vi "UHR-Fleezers Control (host) - 12.5.vi"() -> ()   [LabVIEW 2012] (continued)
  out "error out":errorcluster
  out "error out 2":errorcluster
  in  "Bottom  1 Harvard Syringe Pump Serial Port":refnum<visa-resource-name>="Bottom-Pump1-COM5"
  in  "Center Harvard Syringe Pump Serial Port":refnum<visa-resource-name>="Central-Pump2-COM6"
  in  "Lost Tether Alarm Threshold (pN)":dbl=0.5
  in  "AOM X Cal (nm/MHz)":dbl=155.0
  in  "MCL X Cal (nm/V)":dbl=1070.0
  out "X RF Amplitude Limits (%)":T16={"Minimum"=0.0, "Maximum"=50.0, "Increment"=1.0}
  out "X RF Frequency Limits (MHz)":T16={"Minimum"=60.0, "Maximum"=90.0, "Increment"=1.0}
  out "Y RF Frequency Limits (MHz)":T16={"Minimum"=0.0, "Maximum"=40.0, "Increment"=1.0}
  out "Y RF Amplitude Limits (%)":T16={"Minimum"=0.0, "Maximum"=50.0, "Increment"=1.0}
  in  "Manip. X?":bool=TRUE
  in  "Manip. Y?":bool
  in  "Force Manip Abort":bool
  out "Read cal error":errorcluster
  in  "DAQ Delay (ms)":u32=1000
  in  "Start Scan":bool
  in  "Scan axis":bool=TRUE
  in  "Osc. amp. (V)":dbl=5.0
  in  "Osc. center (V)":dbl=5.0
  in  "Osc. freq. (Hz) 2":dbl=1.0
  in  "MCL Mode":u16(ring) items=["Manual Positioning", "Sinusoidal Wave", "Linear Scan"]
  in  "Begin (V)":dbl
  in  "End (V)":dbl=10.0
  in  "N Points":dbl=20.0
  in  "Delay to Interlace (s)":dbl
  in  "Delayed Interlace Start":bool
  in  "Read Lateness and Rel Phase":bool=TRUE
  out "Vec Mean of T1 T2":dbl[](array[numeric])=[nan, nan]
  in  "Cal read wait (s)":u32=5
  out "Time tether formed":timestamp=timestamp(3419012832.6319866 s since 1904-01-01)
  in  "Sample Chamber Stage Serial Port":refnum<visa-resource-name>="Sample-Stage-COM1"
  in  "Chemyx Syringe Pump Serial Port":refnum<visa-resource-name>="ASRL3::INSTR"
  in  "Limit Min (MHz)":dbl=10.0 caption="Min (MHz)"
  in  "Limit Max (MHz)":dbl=16.0 caption="Max (MHz)"
  in  "Limits Enable":bool=TRUE caption="Enable"
  out "AI labels":string[](array[string])=["T1 Y", "T1 X", "T1 Sum", "T2 Y", "T2 X", "T2 Sum", "T1 FB X", "T1 FB Sum", "T2 FB X", "T2 FB Sum", "PSD Y", "PSD X", "PSD Y Sum"]
  in  "Save Trap Pos. Data":bool=TRUE
  in  "Lower Ch. Cap.":bool
  in  "Top 3 Harvard Syringe Pump Serial Port":refnum<visa-resource-name>="Top-Pump3-COM4"
  out "Database link":path
  out "connection reference":T17
  # "External fluorescence triggering tests:"
  # "After"
  # "During"
  # "Trap On?"
  # "BD Flow ON?"
  # "Samp Flow ON?"
  # "Trap Trig. Fl.?"
  # "Zero It"
  # "Floor it\n(e.g., hp unwinding)"
  # "1"
  # "2"
  # "Fl. Down"
  # "Fl. Up"
  # "Bead sep"
  # "Trap Display:"
  # "APD Display:"
  # "Data Saving"
  # "DAQ"
  # "Trap Manipulation"
  # "Bead Calibration"
  # "Bottom Pump (#1)"
  # "Central Sample Channels"
  # "Top Pump (#3)"
  # "Rate param is ul/h\nVolume param is ul"
  # "Chemyx Pump 2"
  # "Units: \n1 = ml/m\n2 = ml/h\n3 = ul/m\n4 = ul/h"
  # "X"
  # "Amp switch 1st is disabled in the fpga"
  # "Y"
  # "Oscillate Set 1 freq. (debugging)"
  # "BD 1"
  # "BD 2"
  # "AOD Raster Scan"
  # "Approx. trap separations"
  # "X"
  # "Y"
  # "FPGA\nreading"
  # "DMA\ntransfer"
  # "APD Integration Loop"
  # "APD Gates"
  # "APD 2 (Cy5)"
  # "APD 3 (Cy2)"
  # "APD 1 (Cy3)"
  # "X"
  # "2D"
  # "Y"
  # "1D"
  # "Digital Out Control"
  # "Analog Out Control (Feedback Loop)"
  # "Laser Intensity Analog Input"
  # "Operational note:\n\nUse the digital out control to adjust red laser\ntiming (fine tuning).\n\nAt the moment, the red laser analog out\ncontrol timing is identical and set by green \nlaser AO timing (in the same loop).  Otherwise\nyou can not get synchronous timing with the\ncurrent AO expansion board.\n\nSimilarly, the AI measurement is also \nsimultaneous for all three lasers (for the same\nreason).\n\nThese controls are kept for possible future\nuse."
  # "Analog Out Control (Feedback Loop)"
  # "Digital Out Control"
  # "Laser Intensity Analog Input"
  # "Operational note:\n\nThe AI measurement is simultaneous for all three lasers\n(see red laser note).\n\nThese controls are kept for possible future use."
  # "Analog Out Control (Feedback Loop)"
  # "Laser Intensity Analog Input"
  # "Digital Out Control"
  # "Total AI Rates (NOT rates/trap)"
  # "(Samples/trap x Trap Sets)"
  # "(Samples/channel x\n8 if averaging (8 channels)\n4 if no averaging)"
  # "Trap 1"
  # "Trap 2"
  # "Flour./Trap 3"
  # "External Video Window"
  # "MCL Position Debugging"
  # "Temporary Control Storage\n(these used to be somewhere else, still want to keep them)"
  # "Database config"
  # "Y"
  # "X"
  # "Trap Position Difference Limits"
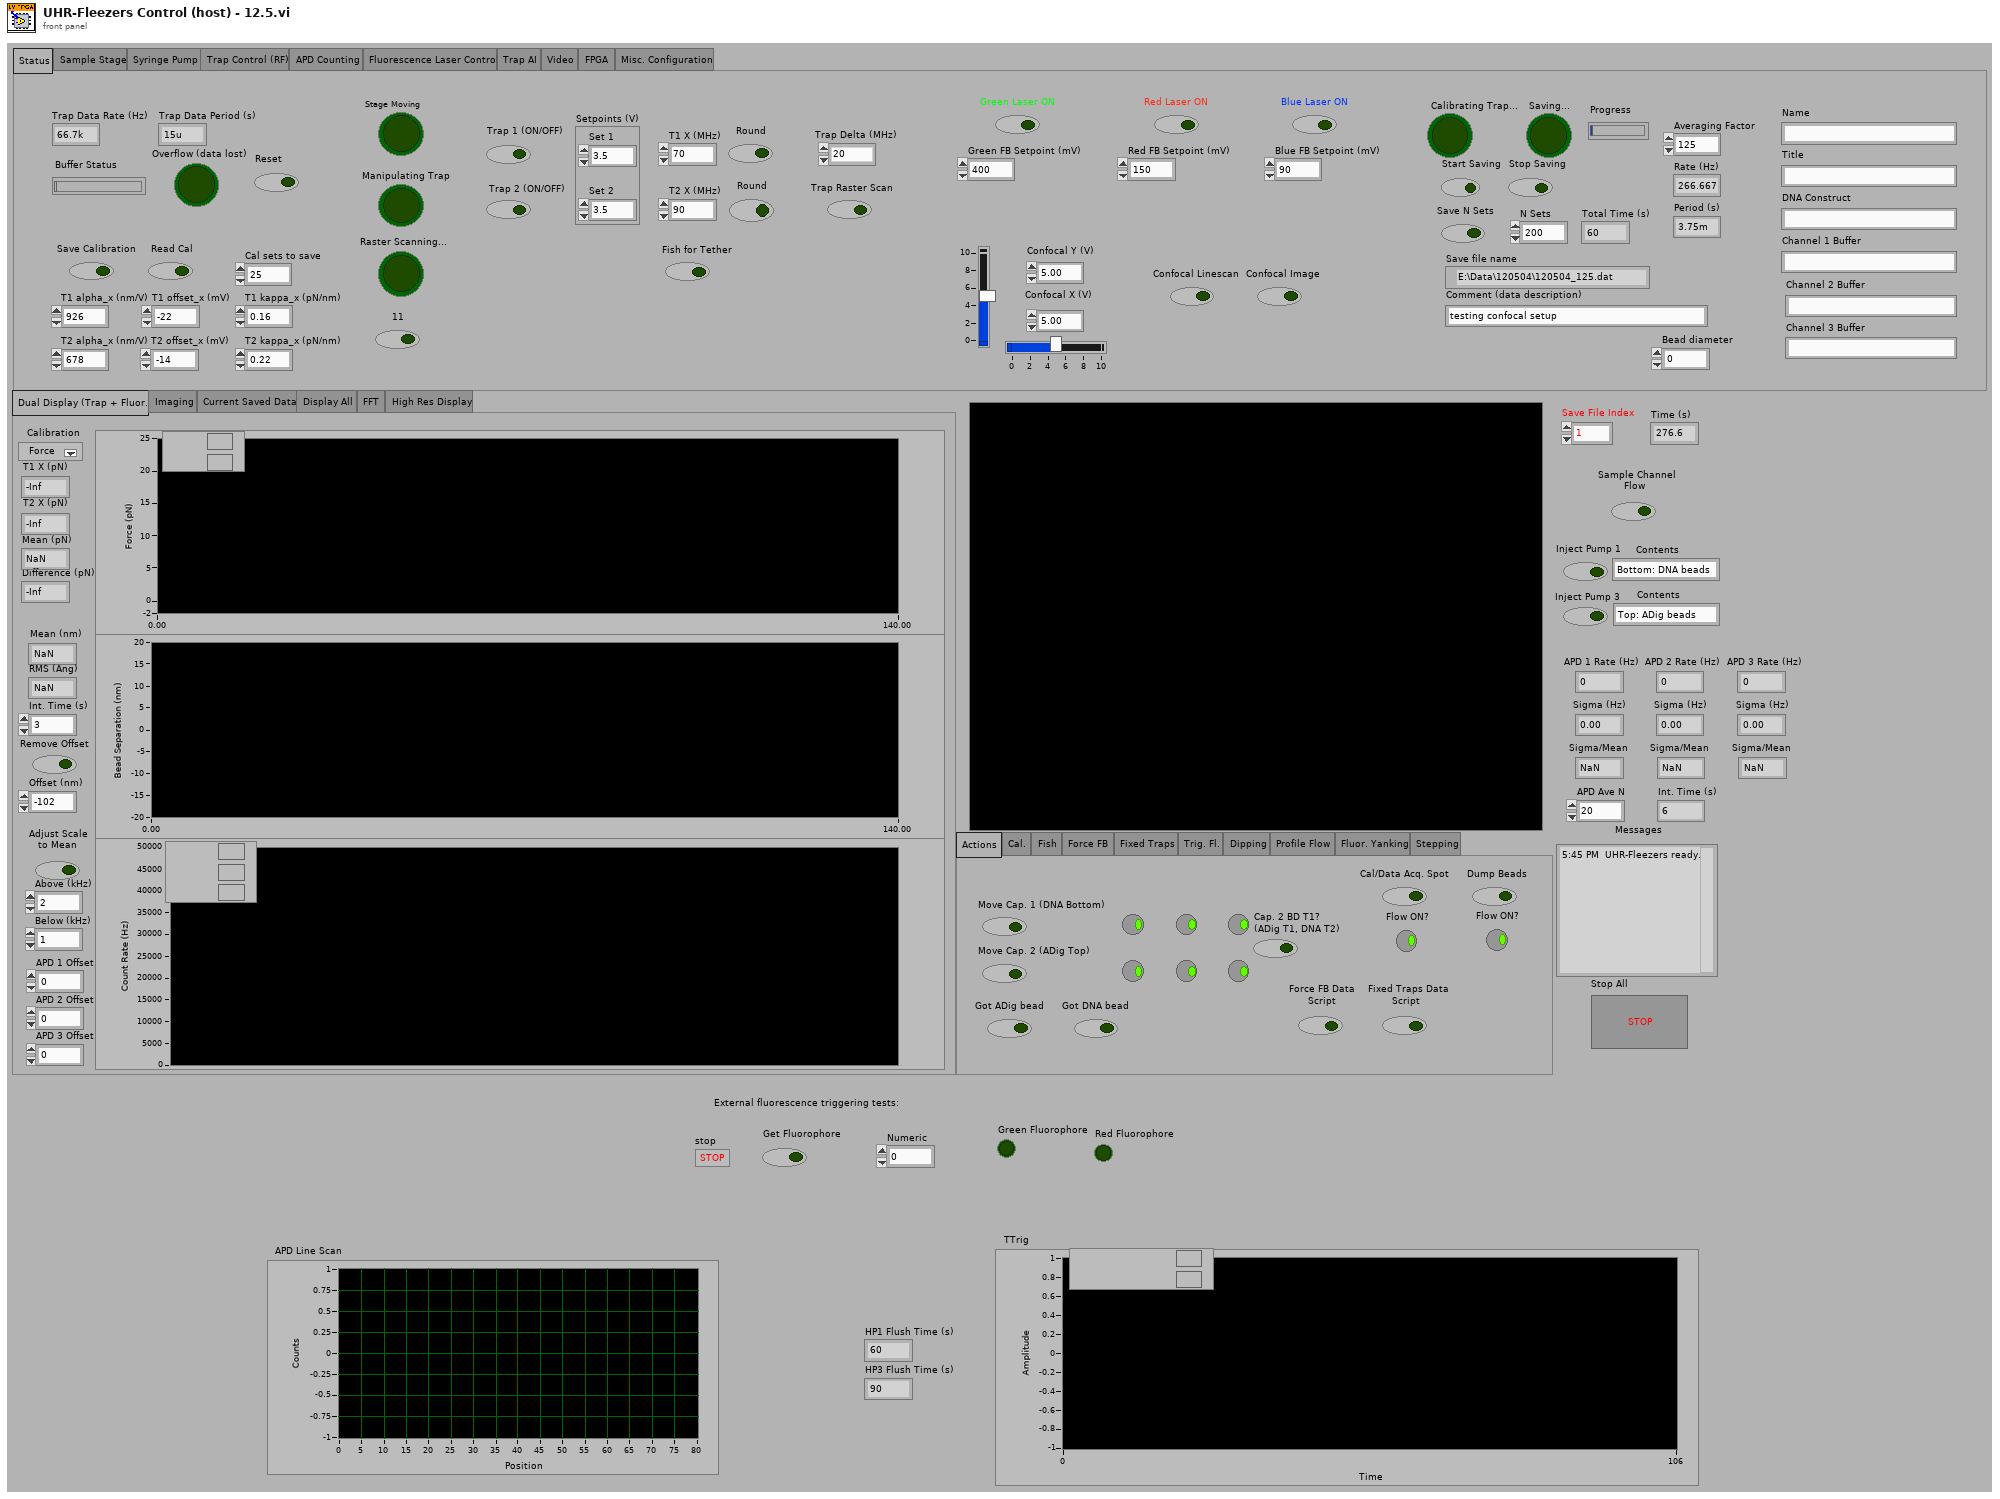
[diagram p1: front panel]
types:
  T1 = enum32{"Actions", "Cal.", "Fish", "Force FB", "Fixed Traps", "Trig. Fl.", "Dipping", "Profile Flow", "Fluor. Yanking", "Stepping"}
  T2 = typedef "IMAQ Image.ctl" = refnum<image>
  T3 = enum32{"Dual Display (Trap + Fluor.)", "Imaging", "Current Saved Data", "Display All", "FFT", "High Res Display"}
  T4 = enum32{"Status", "Sample Stage", "Syringe Pump", "Trap Control (RF)", "APD Counting", "Fluorescence Laser Control", "Trap AI", "Video", "FPGA", "Misc. Configuration"}
  T5 = cluster{"Pump 1":cluster{"Diameter (mm)":dbl, "Units":dbl, "Volume":dbl, "Rate":dbl}, "Pump 2":cluster{"Diameter (mm)":dbl, "Units":dbl, "Volume":dbl, "Rate":dbl}, "Pump 3":cluster{"Diameter (mm)":dbl, "Units":dbl, "Volume":dbl, "Rate":dbl}}
  T6 = enum32{"IR Laser Interlacing (Direct RF Board Control Method)", "AOD Raster Scan", "Feedback on Trap Intensity", "Feedback on Trap Position"}
  T7 = typedef "LVPoint32TypeDef.ctl" = cluster{"Horizontal":i32, "Vertical":i32}
  T8 = cluster{"Scan Range AOD (nm) 2":dbl, "Step Size AOD (nm) 2":dbl, "Scan Speed AOD (nm/s) 2":dbl, "Number of scans (AOD) 2":u16, "Label":string}[]
  T9 = cluster{"proportional gain (Kc)":i16, "integral gain (Kc*Ts/Ti)":i16, "derivative gain (Kc*Td/Ts)":i16}
  T10 = cluster{"Trap 1":fxp<+/-,16,1>, "Trap 2":fxp<+/-,16,1>}
  T11 = cluster{"proportional gain (Kc)":fxp<+/-,16,8>, "integral gain (Kc*Ts/Ti)":fxp<+/-,16,8>, "derivative gain (Kc*Td/Ts)":fxp<+/-,16,8>}
  T12 = cluster{"output high":fxp<+/-,16,1>, "output low":fxp<+/-,16,1>}
  T13 = cluster{"Set 1":fxp<+/-,16,1>, "Set 2":fxp<+/-,16,1>}
  T14 = enum32{"Main Controls", "Green laser (532 nm)", "Red laser (633 nm)", "Blue laser (473 nm)"}
  T15 = cluster{"Set 1":bool, "Set 2":bool, "Set 3":bool}
  T16 = typedef "LVMinMaxIncTypeDef.ctl" = cluster{"Minimum":dbl, "Maximum":dbl, "Increment":dbl}
  T17 = typedef "NI_Database_API.lvlib/Conn ObjectReference.ctl" = refnum<k1>
  T18 = typedef "Image Type" = u32
  T19 = typedef "nirio_resource_hc.ctl" = tag
  T20 = typedef "openfpgaref.8.6.ctl" = refnum<k20>
  T21 = enum16{"empty", "write", "read oldest (queue)", "read newest (stack)", "read all"}
  T22 = cluster{"New Image":T2, "New Image":T2, "New Image":T2, "New Image":T2, "New Image":T2}
  T23 = typedef "XDNodeRunTimeDep.lvlib/timing_clust.ctl" = cluster{"Expected End [f-1]":u64, "Actual End [f-1]":u64, "Finished Late? [f-1]":bool, "Expected End [i-1]":u64, "Actual End [i-1]":u64, "Finished Late? [i-1]":bool, "Expected Start [i]":u64, "Actual Start [i]":u64, "Expected Start [f]":u64, "Actual Start [f]":u64, "Source Name":string, "Structure Name":string, "Period":i64, "Deadline":i64, "Offset":i64, "Start":i64, "Priority":i32, "Timeout":i32, "Mode":T24, "Wakeup Reason":T25, "Error":errorcluster, "Source Type":string, "Secondary Source Type":string, "Global End Time":u64, "Global Start Time":u64, "Frame Duration":u64, "Iteration Duration":u64, "Assigned CPU":i32, "I/O Scan Engine Mode":u32}
  T24 = typedef "XDNodeRunTimeDep.lvlib/nitl_modes.ctl" = enum32{"No Change", "Process missed periods, maintain original phase", "Discard missed periods, maintain original phase", "Process missed periods, ignore original phase", "Discard missed periods, ignore original phase"}
  T25 = typedef "XDNodeRunTimeDep.lvlib/wakeup.ctl" = enum32{"Normal", "Aborted", "Asynchronous wakeup", "Timing source error", "Timed loop error", "Timeout"}
  T26 = enum32{"Status", "Sample Stage", "Syringe Pump", "Trap Control (RF)", "APD Counting", "Fluorescence Laser Control", "Trap AI", "Video", "FPGA"}
  T27 = enum16{"big-endian, network order", "native, host order", "little-endian"}
  T28 = enum16{"open", "replace", "create", "open or create", "replace or create", "replace or create with confirmation"}
  T29 = cluster{"Scan Range AOD (nm) 2":dbl, "Step Size AOD (nm) 2":dbl, "Scan Speed AOD (nm/s) 2":dbl, "Number of scans (AOD) 2":u16, "Label":string}
  T30 = cluster{"[0]":dbl, "[1]":dbl, "[2]":dbl, "[3]":dbl, "[4]":dbl, "[5]":dbl}
  T31 = cluster{"Diameter (mm)":dbl, "Units":dbl, "Volume":dbl, "Rate":dbl}
  T32 = cluster{"Left":i32, "Top":i32, "Width":u32, "Height":u32}
  T33 = cluster{cluster{"Left":i32, "Top":i32, "Width":u32, "Height":u32}}[]
  T34 = enum32{"Normal Display", "Dual Display (APD)", "FFT", "High Res Display"}
  T35 = cluster{"Origin Pixel":cluster{"X":sgl, "Y":sgl}, "Angle Relative to Horizontal (deg)":sgl, "Axis Reference":u32}
  T36 = typedef "Simple Grid Descriptor" = cluster{"X Step":sgl, "Y Step":sgl, "Unit":T37}
  T37 = typedef "Image Unit" = enum32{"Undefined", "Angström", "Micrometer", "Millimeter", "Centimeter", "Meter", "Kilometer", "Microinch", "Inch", "Feet", "Nautical miles", "Standard miles", "Steps"}
  T38 = cluster{"averaging mode":u16, "weighting mode":u16, "number of averages":u32}
  T39 = cluster{"dB On (F)":bool, "unwrap phase (F)":bool, "convert to degree (F)":bool}
  T40 = cluster{string, string, string, string, string, string, string, string}
  T41 = cluster{string, string, string, string, string, string, string, string, string, string, string, string}
  T42 = cluster{string, string, string, string, string, string, string, string, string, string, string, string, string}
  T43 = cluster{string, string, string, string, string, string, string, string, string, string, string, string, string, string}
  T44 = cluster{"BD 1 Frequency 1 (MHz)":dbl, "BD 1 Frequency 2 (MHz)":dbl}
  T45 = cluster{"f0":dbl, "df":dbl, "magnitude":dbl[]}[][]
  T46 = cluster{"Comment (data description)":string, "Channel 1 Buffer":string, "Channel 2 Buffer":string, "Channel 3 Buffer":string, "Title":string, "DNA Construct":string, "Bead diameter":dbl, "Name":string}
  T47 = enum32{"setting", "request", "request control", "info", "statistics", "system settings", "I/O sub system", "HRT control", "camera descriptions", "device specific data", "event sub system settings", "event sub system results", "image memory manager"}
  T48 = typedef "AviRefnum.ctl" = refnum<k1>
  T49 = typedef "imagedata.ctl" = cluster{"image type":i32, "image depth":i32, "image":u8[], "mask":u8[], "colors":u32[], "Rectangle":cluster{"left":i16, "top":i16, "right":i16, "bottom":i16}}
diagram:
  w3 = u16 10 items=["1.0"=10, "1.5"=15, "2.0"=20] ("stop bits (10: 1 bit)")
  w74 = u16 20 items=["1.0"=10, "1.5"=15, "2.0"=20] ("stop bits (10: 1 bit)")
  w77 = u16 20 items=["1.0"=10, "1.5"=15, "2.0"=20] ("stop bits (10: 1 bit)")
  w103 = u16 20 items=["1.0"=10, "1.5"=15, "2.0"=20] ("stop bits (10: 1 bit)")
  w9 = T18 2 items=["Grayscale (U8)", "Grayscale (I16)", "Grayscale (SGL)", "Complex (CSG)", "RGB (U32)", "HSL (U32)", "RGB (U64)", "Grayscale (U16)"] ("Image Type")
  w233 = 10.0 ("y")
  w232 = 32767.0 ("y")
  w248 = 6.0  # clock mult.
  w249 = 49152000.0  # TCXO frequ.
  # "What are these?"
  # "I don't think you need to do this.\nEverytime you want to adjust phase you always set this anyway.\nSince we removed the separate +/- controls.\n\nHaven't added for added fl lasers.  Should remove this code."
  # "Bottom 1 Harvard"
  # "Top 3 Harvard"
  # "Center Harvard"
  # "Bottom 1 Harvard"
  # "Top 3 Harvard"
  # "Center Harvard"
  n1 = Build Array("DIO count 1 (ticks)", "DIO count 2 (ticks)", "DIO count 3 (ticks)") -> (w154:u16[])
  n2 = xnode "Open FPGA VI Reference"("resource name"=T19 "750kHzDAQ") -> ("FPGA VI Reference Out"=w257:T20, "error out"=w256:errorcluster)  [unwired: 1 in]
  n3 = local read "AO1"() -> (w227:dbl)
  n4 = local read "AO2"() -> (w226:dbl)
  n5 = local read "Scan Increment (MHz)"() -> (w244:dbl)
  n6 = local read "Continuous MCL Scanning"() -> (w214:bool)
  n7 = local read "Fast Scan Dir"() -> (w213:bool)
  n8 = xnode "Invoke Method"("FPGA VI Reference In"=w257, "error in"=w256) -> ("FPGA VI Reference Out"=w13:T20, "error out"=w173:errorcluster)
  n9 = local read "Number of scans (MCL)"() -> (w215:u64)
  n10 = Multiply(x=w227, y=w232) -> (x*y=w229:dbl)
  n11 = Multiply(x=w226, y=w232) -> (x*y=w231:dbl)
  n12 = Divide(x=w229, y=w233) -> (x/y=w228:dbl)
  n13 = Divide(x=w231, y=w233) -> (x/y=w230:dbl)
  n14 = To Word Integer(number=w228) -> (16bit integer=w225:i16)
  n15 = To Word Integer(number=w230) -> (16bit integer=w224:i16)
  n16 = Not(x=w213) -> (.not. x?=w208:bool)
  n17 = local read "Cycles/step (MCL)"() -> (w216:u64)
  n18 = Multiply(x=w244, y=1000.0) -> (x*y=w251:dbl)
  n19 = local read "Scan steps (MCL)"() -> (w217:u64)
  n20 = local read "Desired Scan Incr (V)"() -> (w219:dbl)
  n21 = Scale By Power Of 2(n=48, x=w251) -> (x*2^n=w252:dbl)
  n22 = Unbundle By Name(cluster{"output high":i16, "output low":i16} {"output high"=3000, "output low"=0} ("FB output range 1")) -> ("output high"=w55:i16, "output low"=w54:i16)
  n23 = Multiply(x=w249, y=w248) -> (x*y=w247:dbl)
  n24 = Divide(x=w252, y=w247) -> (x/y=w246:dbl)
  n25 = local read "Setpoints (V)"() -> (w263:cluster{"Set 1":dbl, "Set 2":dbl})
  n26 = To Quad Integer(1:w246) -> (0:w243:i64)
  n27 = Divide(x=40000000.0, y="AI Count (ticks)") -> (x/y=w204:dbl)
  n28 = Multiply(x=w219, y=32767.0) -> (x*y=w221:dbl)
  n29 = local read "Trap Intensity PID Gains"() -> (w258:T9)
  n30 = local write "Trap Pos FIFO Timeout"(u16 0 ("Trap Pos FIFO Timeout")) -> ()
  n31 = local read "Number Interlace Sets"() -> (w147:u8)
  n32 = Split 1D Array(array=w154, index=w147) -> (first subarray=w156:u16[])  [unwired: 1 out]
  n33 = Add Array Elements(numeric array=w156) -> (sum=w155:u16)
  n34 = local read "# Samples/channel"() -> (w236:u32)
  n35 = local read "Number of F/B Scans (AOD)"() -> (w237:u16)
  n36 = local read "Not-Interlacing Set"() -> (w146:enum32{"Set 1", "Set 2", "Set 3"})
  n37 = To Unsigned Byte Integer(number=w146) -> (unsigned 8bit integer=w152:u8)
  n38 = Index Array(array=w154, index=w152) -> (element=w153:u16)
  n39 = local read "Feedback On/Off"() -> (w266:cluster{"Set 1":bool, "Set 2":bool})
  n40 = local read "Scan steps (AOD)"() -> (w242:u64)
  n41 = local read "All FB On/Off"() -> (w267:bool)
  n42 = local read "Cycles/step (AOD)"() -> (w241:u64)
  n43 = local write "AI rate (Hz)"(w204) -> ()
  n44 = Divide(x=w221, y=10.0) -> (x/y=w220:dbl)
  n45 = Multiply(x=w242, y=w241) -> (x*y=w240:u64)
  n46 = Unbundle By Name(w258) -> ("proportional gain (Kc)"=w59:i16, "integral gain (Kc*Ts/Ti)"=w58:i16, "derivative gain (Kc*Td/Ts)"=w57:i16)
  n47 = property on="AI Count (ticks)" class="DigNum (strict)"("Val(Sgnl)"="AI Count (ticks)") -> ()  [unwired: 2 in, 2 out]
  n48 = Multiply(x=3276.7, y=w263) -> (x*y=w262:cluster{"Set 1":dbl, "Set 2":dbl})
  n49 = To Word Integer(number=w220) -> (16bit integer=w218:i16)
  n50 = Multiply(x=w240, y=u64 2) -> (x*y=w238:u64)
  n51 = Divide(x=w204, y="FPGA Ave.") -> (x/y=w205:dbl)
  n52 = To Word Integer(number=w262) -> (16bit integer=w261:cluster{"Set 1":i16, "Set 2":i16})
  n53 = Multiply(x=w238, y=w237) -> (x*y=w235:u64)
  n54 = local read "Sets to FIFO (Traps)"() -> (w63:T15)
  n55 = local write "Ave. Rate (Hz)"(w205) -> ()
  n56 = Divide(x=w235, y=w236) -> (x/y=w234:dbl)
  n57 = Unbundle By Name(w261) -> ("Set 1"=w260:i16, "Set 2"=w259:i16)
  n58 = local read "2D or 1D Scan"() -> (w165:bool)
  n59 = local write "Data points/scans"(w235) -> ()
  n60 = local read "Scan BD"() -> (w253:bool)
  n61 = And(x=w266, y=w267) -> (x .and. y?=w265:cluster{"Set 1":bool, "Set 2":bool})
  n62 = local write "Data points/scan (f/b)"(w238) -> ()
  n63 = Reciprocal(x=w205) -> (1/x=w206:dbl)
  n64 = local read "N Acq Sets (Traps + Fl.)"() -> (w197:i16)
  n65 = local write "N sets should be saved"(w234) -> ()
  n66 = Unbundle By Name(w265) -> ("Set 1"=w269:bool, "Set 2"=w268:bool)
  n67 = local read "Interlace"() -> (w148:bool)
  n68 = Select(t=w155, s=w148, f=w153) -> (s? t:f=w145:u16)
  n69 = local write "Update Count (MCL)"(w145) -> ()
  n70 = local write "Total Counts (ticks)"(w145) -> ()
  n71 = local write "Ave. Period (s)"(w206) -> ()
  n72 = Unbundle By Name(w63) -> ("Set 1"=w62:bool, "Set 2"=w61:bool, "Set 3"=w60:bool)
  n73 = property on="2D or 1D Scan" class="Bool (strict)"("Val(Sgnl)"=w165) -> ()  [unwired: 2 in, 2 out]
  n74 = xnode "Read/Write Control"("FPGA VI Reference In"=w164, "error in"=w173, "ai count"="AI Count (ticks)", "Interlace ON/OFF"=w148, "Number Interlace Cycles"=w147, "Set 1"=w62, "Set 2"=w61, "Set 3"=w60, "FB On/Off Set 1"=w269, "FB On/Off Set 2"=w268, "Interlace Off Parameters"=w146, "FB Setpoint Set 1"=w260, "FB Setpoint Set 2"=w259, "P1"=w59, "I1"=w58, "D1"=w57, "FB1 output high"=w55, "FB1 output low"=w54, "Cycles per step"=w241, "Scan BD"=w253, "Number of scans"=w237, "Scan steps"=w242, "Scan freq.  increment"=w243, "AO1"=w225, "AO2"=w224, "Scan freq.  increment (MCL)"=w218, "Scan steps (MCL)"=w217, "Cycles per step (MCL)"=w216, "Number of scans (MCL)"=w215, "MCL count"=w145, "Cont. Scan (MCL)"=w214, "MCL Scan Axis"=w208, "1D or 2D Scan?"=w165, "N of AI1 Int Acq Sets"=w197, "Amp switch delay"="Amp switch delay", "Swap F1 and F2"="Swap F1 and F2", "APD to FIFO"=FALSE, "DIO count 1 (ticks)"="DIO count 1 (ticks)", "DIO count 2 (ticks)"="DIO count 2 (ticks)", "DIO count 3 (ticks)"="DIO count 3 (ticks)") -> ("FPGA VI Reference Out"=w15:T20, "error out"=w14:errorcluster)  [unwired: 1 in]
  n75 = local read "Laser interlacing mode"() -> (w144:enum32{"Laser ON", "Laser OFF", "Interlace"})
  n76 = local read "Green Laser ON"() -> (w143:bool)
  n77 = local read "Trap Pos. FB Range"() -> (w53:T12)
  n78 = local read "Trap Pos. FB Gains"() -> (w52:T11)
  n79 = Multiply(x="Green Intensity % (FB OFF)", y=655.35) -> (x*y=w136:dbl)
  n80 = local read "Invert laser interlacing"() -> (w30:bool)
  n81 = local read "Trap Pos. AI1 X Pre-scale"() -> (w91:u16)
  n82 = Multiply(x="Green FB Setpoint (mV)", y=3.2767) -> (x*y=w133:dbl)
  n83 = local read "Trap Pos FB Int Count"() -> (w85:u16)
  n84 = local read "Differential FB?"() -> (w79:bool)
  n85 = local read "Neg. TTrig FPGA"() -> (w81:bool)
  n86 = Multiply(x="Red FB Setpoint (mV)", y=3.2767) -> (x*y=w39:dbl)
  n87 = To Unsigned Word Integer(number=w136) -> (unsigned 16bit integer=w134:u16)
  n88 = Multiply(x="Red Intensity % (FB OFF)", y=655.35) -> (x*y=w35:dbl)
  n89 = To Word Integer(number=w133) -> (16bit integer=w131:i16)
  n90 = Unbundle By Name("Green FB Gains") -> ("proportional gain (Kc)"=w44:i16, "integral gain (Kc*Ts/Ti)"=w43:i16, "derivative gain (Kc*Td/Ts)"=w42:i16)
  n91 = case shown="False" w143 {
    tunnel: w144 -> [_ w295]
    tunnel: [enum32{"Laser ON", "Laser OFF", "Interlace"}."Laser OFF" ("Green laser mode") w295] -> w29
    frame False {
    }
    frame True {
    }
  }
  n92 = To Word Integer(number=w39) -> (16bit integer=w36:i16)
  n93 = Unbundle By Name("Red FB Gains") -> ("proportional gain (Kc)"=w27:i16, "integral gain (Kc*Ts/Ti)"=w26:i16, "derivative gain (Kc*Td/Ts)"=w25:i16)
  n94 = Unbundle By Name(w52) -> ("proportional gain (Kc)"=w48:fxp<+/-,16,8>, "integral gain (Kc*Ts/Ti)"=w47:fxp<+/-,16,8>, "derivative gain (Kc*Td/Ts)"=w46:fxp<+/-,16,8>)
  n95 = To Unsigned Word Integer(number=w35) -> (unsigned 16bit integer=w32:u16)
  n96 = Unbundle By Name(w53) -> ("output high"=w51:fxp<+/-,16,1>, "output low"=w49:fxp<+/-,16,1>)
  n97 = local read "Trap Pos FB Monitor\nT1 or T2"() -> (w96:bool)
  n98 = local read "Trap Pos FB Negate Action"() -> (w95:bool)
  n99 = local read "Trap Pos. FB Offset Factor"() -> (w94:i64)
  n100 = local read "Trap Pos. FB Mult Factor"() -> (w93:i64)
  n101 = xnode "Read/Write Control"("FPGA VI Reference In"=w15, "error in"=w14, "Invert GI 2"=w30, "Operating Mode 2"=w29, "P3"=w44, "I3"=w43, "D3"=w42, "Green FB Setpoint"=w131, "Green FB On/Off"="Green FB On/Off", "Current Out"=w134, "Green int current ON count adj"="Green int current ON count adj", "Operating Mode"=w29, "Invert GI"=w30, "Trap Pos FB Monitor T1 or T2"=w96, "Trap Pos FB Negate Action"=w95, "Trap Pos. FB Offset Factor"=w94, "Trap Pos. FB Mult Factor"=w93, "Force feedback"=FALSE, "AI1 X Scale"=w91, "Trap Pos to FIFO"=TRUE, "Trap Pos FB Int Count"=w85, "TTrig Negate Pos"=w81, "FB Trig Integrate"="FB Trig Integrate", "Diff FB Measurement?"=w79, "Negate Diff?"="Negate Diff?", "P2"=w48, "I2"=w47, "D2"=w46, "FB2 output high"=w51, "FB2 output low"=w49, "Red FB Setpoint"=w36, "RI Current Out"=w32, "Red int current ON count adj"="Red int current ON count adj", "Red Laser Operating Mode"=w29, "RI Operating Mode 2"=w29, "Invert RI 2"=w30, "Invert RI"=w30, "P4"=w27, "I4"=w26, "D4"=w25, "Red FB On/Off"="Red FB On/Off") -> ("FPGA VI Reference Out"=w20:T20, "error out"=w22:errorcluster)
  n102 = stacked-sequence {
    tunnel: w22 -> [_ _ _ w306]
    tunnel: [_ _ _ w306] -> w21
    tunnel: w20 -> [_ _ _ w307]
    tunnel: [_ _ _ w307] -> w19
    frame #0 {
      w296 = T21."empty" ("mode")
      # "Clear external fluorescence triggering FIFO"
      # "APD loop counts"
      # "Fluorescence loop counts (rates)"
      n103 = local read "APD Integration Time (s)"() -> (w298:dbl)
      n104 = local read "Interlace ON count"() -> (w299:u16)
      n105 = call "Smart Buffer (DBL) 1.vi"("mode"=w296) -> ()  [unwired: 5 in, 6 out]
      n106 = call "Smart Buffer (DBL) 2.vi"("mode"=w296) -> ()  [unwired: 5 in, 6 out]
      n107 = property on="APD Integration Time (s)" class="DigNum (strict)"("Val(Sgnl)"=w298) -> ()  [unwired: 2 in, 2 out]
      n108 = property on="Interlace ON count" class="DigNum (strict)"("Val(Sgnl)"=w299) -> ()  [unwired: 2 in, 2 out]
      "Number of APDs" <- 3.0 ("Number of APDs")
    }
    frame #1 {
      # "Number of APDs affects\nAPD DMA transfer"
      # "General settings for all lasers:"
      # "And includes all laser\nON/OFF settings"
      # "Fluorescent lasers settings:"
      # "Blue laser settings:"
      n109 = local read "Laser interlacing mode"() -> (w301:enum32{"Laser ON", "Laser OFF", "Interlace"})
      n110 = local read "Invert laser interlacing"() -> (w300:bool)
      n111 = local read "Blue FB On/Off"() -> (w302:bool)
      n112 = property on="Blue FB On/Off" class="Bool (strict)"("Val(Sgnl)"=w302) -> ()  [unwired: 2 in, 2 out]
      n113 = property on="Invert laser interlacing" class="Bool (strict)"("Val(Sgnl)"=w300) -> ()  [unwired: 2 in, 2 out]
      n114 = property on="Laser interlacing mode" class="RadioBtnsControl (strict)"("Val(Sgnl)"=w301) -> ()  [unwired: 2 in, 2 out]
    }
    frame #2 {
      w303 = path "C:/Home/wheeler/Comstock-LabView-Link.udl" ("connection information")
      # "Initialize the database connection"
      n115 = call-poly <vilib>:"DB Tools Open Connection.vi"("connection information"=w303) -> ("connection reference"=w304:T17)  [unwired: 7 in, 1 out]
      "connection reference" <- w304
      n116 = local write "connection reference"(w304) -> ()
      n117 = local write "Database link"(w303) -> ()
    }
    frame #3 {
      n118 = Wait (ms)(milliseconds to wait=u32 1000) -> ()  [unwired: 1 out]
    }
  }
  n119 = local write "Offset (nm)"(0.0 ("Offset (nm)")) -> ()
  n120 = local write "Bead Mean (nm)"(0.0 ("Bead Mean (nm)")) -> ()
  n121 = xnode "Invoke Method"("FPGA VI Reference In"=w19, "error in"=w21, "Requested Depth"="Trap AI FIFO Depth") -> ("FPGA VI Reference Out"=w99:T20, "error out"=w98:errorcluster)  [unwired: 1 out]
  n122 = xnode "Invoke Method"("FPGA VI Reference In"=w99, "error in"=w98, "Requested Depth"="Trap Position FIFO Depth") -> ("FPGA VI Reference Out"=w87:T20, "error out"=w86:errorcluster)  [unwired: 1 out]
  n123 = flat-sequence "Safety limits on RF frequencies and amplitudes (for AOM protection)" {
    tunnel: w13 -> [w312]
    tunnel: [w312] -> w164
    tunnel: [w311] -> w163
    tunnel: [w310] -> w162
    tunnel: [w308] -> w160
    tunnel: [w309] -> w161
    frame #0 {
      w309 = T16 {"Minimum"=0.0, "Maximum"=40.0, "Increment"=1.0} ("Min Max Inc")
      w308 = T16 {"Minimum"=0.0, "Maximum"=50.0, "Increment"=1.0} ("Data Entry Limits")
      w311 = T16 {"Minimum"=60.0, "Maximum"=90.0, "Increment"=1.0} ("Min Max Inc")
      w310 = T16 {"Minimum"=0.0, "Maximum"=50.0, "Increment"=1.0} ("Data Entry Limits")
      n124 = property on="BD 2 Frequency 1 (MHz)" class="DigNum (strict)"("Data Range"=w309) -> ()  [unwired: 2 in, 2 out]
      n125 = property on="BD 2 Frequency 3 (MHz)" class="DigNum (strict)"("Data Range"=w309) -> ()  [unwired: 2 in, 2 out]
      n126 = property on="BD 2 Frequency 2 (MHz)" class="DigNum (strict)"("Data Range"=w309) -> ()  [unwired: 2 in, 2 out]
      n127 = property on="BD 1 Frequency 1 (MHz)" class="DigNum (strict)"("Data Range"=w311) -> ()  [unwired: 2 in, 2 out]
      n128 = property on="BD 1 Frequency 2 (MHz)" class="DigNum (strict)"("Data Range"=w311) -> ()  [unwired: 2 in, 2 out]
      n129 = property on="BD 1 Frequency 3 (MHz)" class="DigNum (strict)"("Data Range"=w311) -> ()  [unwired: 2 in, 2 out]
      n130 = property on="BD 2 Amplitude 1 (%)" class="DigNum (strict)"("Data Range"=w308) -> ()  [unwired: 2 in, 2 out]
      n131 = property on="BD 2 Amplitude 2 (%)" class="DigNum (strict)"("Data Range"=w308) -> ()  [unwired: 2 in, 2 out]
      n132 = property on="BD 2 Amplitude 3 (%)" class="DigNum (strict)"("Data Range"=w308) -> ()  [unwired: 2 in, 2 out]
      n133 = property on="BD 1 Amplitude 3 (%)" class="DigNum (strict)"("Data Range"=w310) -> ()  [unwired: 2 in, 2 out]
      n134 = property on="BD 1 Amplitude 2 (%)" class="DigNum (strict)"("Data Range"=w310) -> ()  [unwired: 2 in, 2 out]
      n135 = property on="BD 1 Amplitude 1 (%)" class="DigNum (strict)"("Data Range"=w310) -> ()  [unwired: 2 in, 2 out]
      "X RF Frequency Limits (MHz)" <- w311
      "X RF Amplitude Limits (%)" <- w310
      "Y RF Amplitude Limits (%)" <- w308
      "Y RF Frequency Limits (MHz)" <- w309
    }
  }
  n136 = xnode "Invoke Method"("FPGA VI Reference In"=w87, "error in"=w86) -> ("FPGA VI Reference Out"=w172:T20, "error out"=w171:errorcluster)  [unwired: 1 in]
  n137 = flat-sequence "Initial FPGA Loop Relative Phase Adjustment" {
    tunnel: "Initial Phase Adjustment (AI1)" -> [w330]
    tunnel: "Initial Phase Adjustment (GI)" -> [w329]
    tunnel: w172 -> [w328]
    tunnel: w171 -> [w327]
    tunnel: "Initial Phase Adj. (MCL)" -> [w326]
    tunnel: [w331] -> w181
    tunnel: [w325] -> w177
    tunnel: "Initial Phase Adjustment (APD Acq)" -> [w324]
    tunnel: "Initial Phase Adjustment (APD 1 Gate)" -> [w323]
    tunnel: "Initial Phase Adjustment (Green FB)" -> [w322]
    tunnel: "Initial Phase Adjustment (GI) 2" -> [w321]
    tunnel: "Initial Phase Adjustment (APD 2 Gate)" -> [w320]
    tunnel: "Initial Phase Adjustment (RI)" -> [w319]
    tunnel: "Initial Phase Adjustment (RI) 2" -> [w318]
    tunnel: "Initial Phase Adjustment (RI FB)" -> [w317]
    tunnel: "Initial Phase Adjustment (BI DO)" -> [w316]
    tunnel: "Initial Phase Adjustment (BI AO)" -> [w315]
    tunnel: "Initial Phase Adjustment (BI AI)" -> [w314]
    tunnel: "Initial Phase Adjustment (APD 3 Gate)" -> [w313]
    tunnel: w181 -> [w333]
    tunnel: [w334] -> w178
    tunnel: w177 -> [w334]
    tunnel: [w333] -> w176
    tunnel: w178 -> [w337]
    tunnel: w176 -> [w336]
    tunnel: [w339] -> w175
    tunnel: [w338] -> w174
    tunnel: [w341] -> w179
    tunnel: [w342] -> w180
    tunnel: w175 -> [w342]
    tunnel: w174 -> [w341]
    frame #0 {
      n138 = xnode "Read/Write Control"("FPGA VI Reference In"=w328, "error in"=w327, "Phase count adjustment"=w330, "Phase count adjustment (GI)"=w329, "Phase count adjustment (MCL)"=w326, "Phase Count Adjustment (APD Acq)"=w324, "Phase count adjustment (APD 1 Gate)"=w323, "Phase count adjustment (APD 2 Gate)"=w320, "Phase count adjustment (Green FB)"=w322, "Phase count adjustment (GI) 2"=w321, "Phase count adjustment (RI)"=w319, "Phase count adjustment (RI) 2"=w318, "Phase count adjustment (Red FB)"=w317, "Phase count adjustment (BI AO)"=w315, "Phase count adjustment (BI D)"=w316, "Phase count adjustment (Blue Int)"=w314, "Phase count adjustment (APD 3 Gate)"=w313) -> ("FPGA VI Reference Out"=w325:T20, "error out"=w331:errorcluster)
    }
    frame #1 {
      n139 = Wait (ms)(milliseconds to wait=u32 100) -> ()  [unwired: 1 out]
    }
    frame #2 {
      w335 = TRUE
      n140 = xnode "Read/Write Control"("FPGA VI Reference In"=w337, "error in"=w336, "+ phase"=w335, "+ phase (GI)"=w335, "+ phase (MCL)"=w335, "+ phase (APD Acq)"=w335, "+ phase (APD 1 Gate)"=w335, "+ phase (APD 2 Gate)"=w335, "+ phase (Green FB)"=w335, "+ phase (GI) 2"=w335, "+ phase (RI)"=w335, "+ phase (RI) 2"=w335, "+ phase (BI AO)"=w335, "+ phase (BI D)"=w335, "+ phase (Blue Int)"=w335, "+ phase (APD 3 Gate)"=w335) -> ("FPGA VI Reference Out"=w338:T20, "error out"=w339:errorcluster)
    }
    frame #3 {
      n141 = Wait (ms)(milliseconds to wait=u32 100) -> ()  [unwired: 1 out]
    }
  }
  n142 = local read "Phase adj. (Green FB)"() -> (w157:i16)
  n143 = local read "Phase adj. (GI) 2"() -> (w137:i16)
  n144 = local read "Phase adjust (MCL)"() -> (w209:i16)
  n145 = local read "Phase adj. (AI1)"() -> (w211:i16)
  n146 = local read "Phase adj. (GI)"() -> (w210:i16)
  n147 = xnode "Read/Write Control"("FPGA VI Reference In"=w179, "error in"=w180, "Phase count adjustment"=w211, "Phase count adjustment (GI)"=w210, "Phase count adjustment (MCL)"=w209, "Phase Count Adjustment (APD Acq)"="Phase Adj. (APD Acq)", "Phase count adjustment (APD 1 Gate)"="Phase Adj. (APD 1 Gate)", "Phase count adjustment (APD 2 Gate)"="Phase Adj. (APD 2 Gate)", "Phase count adjustment (Green FB)"=w157, "Phase count adjustment (GI) 2"=w137) -> ("FPGA VI Reference Out"=w123:T20, "error out"=w186:errorcluster)
  n148 = call "Initialize RF boards - interlace 3.vi"("error in"=w186, "FPGA VI Reference In"=w123) -> ("error out"=w184:errorcluster, "FPGA VI Reference Out"=w185:T20)
  n149 = call "set RF board frequency - interlace.vi"("Board 2 Frequency Limits"=w161, "Board 1 Frequency Limits"=w163, "error in"=w184, "FPGA VI Reference In"=w185, "Board 2 Frequency 3 (MHz)"="BD 2 Frequency 3 (MHz)", "Board 1 Frequency 3 (MHz)"="BD 1 Frequency 3 (MHz)", "Board 2 Frequency 2 (MHz)"="BD 2 Frequency 2 (MHz)", "Board 2 Frequency 1 (MHz)"="BD 2 Frequency 1 (MHz)", "Board 1 Frequency 2 (MHz)"="BD 1 Frequency 2 (MHz)", "Board 1 Frequency 1  (MHz)"="BD 1 Frequency 1 (MHz)") -> ("error out"=w284:errorcluster, "FPGA VI Reference Out"=w285:T20)
  n150 = call "set RF board amplitude - interlace.vi"("Board 2 Amplitude Limits"=w160, "Board 1 Amplitude Limits"=w162, "error in"=w284, "FPGA VI Reference In"=w285, "Board 2 Amplitude 3 (%)"="BD 2 Amplitude 3 (%)", "Board 1 Amplitude 3 (%)"="BD 1 Amplitude 3 (%)", "Board 2 Amplitude 2 (%)"="BD 2 Amplitude 2 (%)", "Board 2 Amplitude 1 (%)"="BD 2 Amplitude 1 (%)", "Board 1 Amplitude 2 (%)"="BD 1 Amplitude 2 (%)", "Board 1 Amplitude 1 (%)"="BD 1 Amplitude 1 (%)") -> ("error out"=w272:errorcluster, "FPGA VI Reference Out"=w273:T20)
  n151 = flat-sequence {
    tunnel: w273 -> [w352]
    tunnel: w272 -> [w351]
    tunnel: [w350] -> w277
    tunnel: [w349] -> w276
    tunnel: [w356] -> w275
    tunnel: w277 -> [w356]
    tunnel: [w355] -> w274
    tunnel: w276 -> [w355]
    tunnel: w275 -> [w365]
    tunnel: w274 -> [w364]
    tunnel: [w363] -> w12
    tunnel: [w362] -> w88
    frame #0 {
      w343 = FALSE ("Retract Pump 3")
      n152 = local read "Trap 1 (ON/OFF)"() -> (w344:bool)
      n153 = xnode "Read/Write Control"("FPGA VI Reference In"=w352, "error in"=w351, "Direct RF Box  Communication"=FALSE) -> ("FPGA VI Reference Out"=w350:T20, "error out"=w349:errorcluster)
      n154 = local write "Saving..."(FALSE ("Saving Data")) -> ()
      n155 = local write "Stop All"(FALSE ("Stop All")) -> ()
      n156 = local write "Retract Pump 1"(w343) -> ()
      n157 = local write "Retract Pump 3"(w343) -> ()
      n158 = local write "Index"(1.0 ("Index")) -> ()
      n159 = property on="Trap 1 ON" class="Bool (strict)"("Value"=w344) -> ()  [unwired: 2 in, 2 out]
      "Manipulating Trap" <- FALSE ("Manipulating Trap")
    }
    frame #1 {
      n160 = local read "Trap 2 (ON/OFF)"() -> (w354:bool)
      n161 = Wait (ms)(milliseconds to wait=u32 10) -> ()  [unwired: 1 out]
      n162 = property on="Trap 2 ON" class="Bool (strict)"("Val(Sgnl)"=w354) -> ()  [unwired: 2 in, 2 out]
    }
    frame #2 {
      n163 = local read "Scan Range (nm)"() -> (w358:dbl)
      n164 = xnode "Read/Write Control"("FPGA VI Reference In"=w365, "error in"=w364, "FPGA Controls  RF Box"=TRUE ("Direct RF Box  Communication")) -> ("FPGA VI Reference Out"=w363:T20, "error out"=w362:errorcluster)
      n165 = call "Update messages.vi"("Message to add"="UHR-Fleezers ready.", "Old message string"="") -> ("New message string"=w361:string)
      n166 = local write "Messages"(w361) -> ()
      n167 = property on="Scan Range (nm)" class="DigNum (strict)"("Val(Sgnl)"=w358) -> ()  [unwired: 2 in, 2 out]
    }
  }
  n168 = Subtract(x="BD 1 Frequency 1 (MHz)", y="BD 1 Frequency 2 (MHz)") -> (x-y=w196:dbl)
  n169 = Subtract(x="BD 2 Frequency 1 (MHz)", y="BD 2 Frequency 2 (MHz)") -> (x-y=w195:dbl)
  n170 = Square(x=w195) -> (x^2=w193:dbl)
  n171 = Square(x=w196) -> (x^2=w194:dbl)
  n172 = Add(x=w194, y=w193) -> (x+y=w192:dbl)
  n173 = Square Root(x=w192) -> (sqrt(x)=w191:dbl)
  n174 = local write "Trap Delta (MHz)"(w191) -> ()
  n175 = call-poly "VISA Configure Serial Port"("VISA resource name"="VISA resource name", "baud rate (9600)"=u32 115200, "stop bits (10: 1 bit)"=w3) -> ("VISA resource name out"=w2:refnum<visa-resource-name>, "error out"=w1:errorcluster)  [unwired: 4 in, 7 out]
  n176 = call-poly "VISA Configure Serial Port"("VISA resource name"="Bottom  1 Harvard Syringe Pump Serial Port", "baud rate (9600)"=u32 115200, "stop bits (10: 1 bit)"=w74) -> ("VISA resource name out"=w70:refnum<visa-resource-name>, "error out"=w69:errorcluster)  [unwired: 4 in, 7 out]
  n177 = call-poly "VISA Configure Serial Port"("VISA resource name"="Top 3 Harvard Syringe Pump Serial Port", "baud rate (9600)"=u32 115200, "stop bits (10: 1 bit)"=w77) -> ("VISA resource name out"=w72:refnum<visa-resource-name>, "error out"=w71:errorcluster)  [unwired: 4 in, 7 out]
  n178 = call-poly "VISA Configure Serial Port"("VISA resource name"="Sample Chamber Stage Serial Port") -> ("VISA resource name out"=w118:refnum<visa-resource-name>, "error out"=w119:errorcluster)  [unwired: 5 in, 8 out]
  "Stage Control Serial Error" <- w119
  n179 = local write "Blue Error Out"(w1) -> ()
  n180 = call-poly "VISA Configure Serial Port"("VISA resource name"="Center Harvard Syringe Pump Serial Port", "baud rate (9600)"=u32 115200, "stop bits (10: 1 bit)"=w103) -> ("VISA resource name out"=w100:refnum<visa-resource-name>, "error out"=w101:errorcluster)  [unwired: 4 in, 7 out]
  n181 = call "IMAQ Create"("Image Name"="APD 1 Image", "Image Type"=w9) -> ("New Image"=w109:T2)  [unwired: 3 in, 1 out]
  n182 = call "IMAQ Create"("Image Name"="APD 2 Image", "Image Type"=w9) -> ("New Image"=w108:T2)  [unwired: 3 in, 1 out]
  n183 = call "IMAQ Create"("Image Name"="APD 3 Image", "Image Type"=w9) -> ("New Image"=w8:T2)  [unwired: 3 in, 1 out]
  n184 = call "IMAQ Create"("Image Name"="Det. X Image", "Image Type"=w9) -> ("New Image"=w107:T2)  [unwired: 3 in, 1 out]
  n185 = call "IMAQ Create"("Image Name"="Det. Y Image", "Image Type"=w9) -> ("New Image"=w106:T2)  [unwired: 3 in, 1 out]
  n186 = Bundle("New Image"=w109, "New Image"=w108, "New Image"=w8, "New Image"=w107, "New Image"=w106) -> (w105:T22)  [unwired: 1 in]
  n187 = node-c288(3 ("Processor")) -> (w125:T23)  [unwired: 3 out]
  n188 = node-c288() -> (w114:T23)  [unwired: 4 in]
  n189 = node-c288(2 ("Processor")) -> (w127:T23)  [unwired: 3 out]
  n190 = node-c288() -> (w129:T23)  [unwired: 4 out]
  n191 = node-c288(i64 1 ("Period"), 1 ("Processor")) -> (w200:T23)  [unwired: 2 out]
  n192 = node-c288() -> (w7:T23)  [unwired: 4 out]
  n193 = timed-loop "Oscillate Trap/AOM (fishing, conjugate plane alignment)" {
    tunnel: w13 -> [w368]
    tunnel: [w367] -> w130
    timing: w125 -> [_]
    timing-out: [_] -> w124
    stop <- w367 stop-if-true
    n194 = node-c288() -> ()  [unwired: 2 out]
    n195 = event shown="[1] \"Fl. Triggered...\": Value Change" {
      selector: _ -> [_ _ _]
      dyn-events: _ -> [_ _ _]
      timeout: _ -> [_ _ _]
      tunnel: w368 -> [w375 _ _]
      tunnel: [FALSE ("Stop All") _ w964] -> w367
      event "Oscillate Set 1", "Fish for Tether": Value Change {
        n196 = event-data() -> ()  [unwired: 6 out]
        n197 = local read "Oscillate Set 1"() -> (w374:bool)
        n198 = Or(x=w374, y="Fish for Tether") -> (x .or. y?=w372:bool)
        n199 = case shown="True" w372 {
          tunnel: w375 -> [_ w378]
          tunnel: "Fish for Tether" -> [_ w377]
          frame False {
          }
          frame True {
            n200 = case shown="True" w377 {
              selector: w377 -> [w381 w387]
              tunnel: [w381 w387] -> w376
              frame False {
              }
              frame True {
                n201 = local write "Scan axis 2"(TRUE) -> ()
                n202 = local write "Tether"(FALSE ("Tether")) -> ()
                n203 = local read "Flow ON during cal?"() -> (w382:bool)
                n204 = property on="Trap Delta (MHz)" class="DigNum (strict)"("Val(Sgnl)"="Furthest Delta (MHz)") -> ()  [unwired: 2 in, 2 out]
                n205 = Or(x="Flow ON during \nfishing?", y=w382) -> (x .or. y?=w383:bool)
                n206 = Wait (ms)(milliseconds to wait=u32 500) -> ()  [unwired: 1 out]
                n207 = property on="Sample Channel\nFlow" class="Bool (strict)"("Val(Sgnl)"=w383) -> ()  [unwired: 2 in, 2 out]
              }
            }
            n208 = node-c288() -> (w380:T23)  [unwired: 4 out]
            n209 = timed-loop "Oscillate AOD" {
              timing: w380 -> [_]
              timing-out: [_] -> w379
              tunnel: w378 -> [w397]
              tunnel: w376 -> [w390]
              i -> [w399]
              stop <- w396 stop-if-true
              n210 = node-c288() -> (w398:i64)  [unwired: 1 out]
              n211 = flat-sequence {
                tunnel: w399 -> [w426]
                tunnel: w398 -> [w425]
                tunnel: w397 -> [w404]
                tunnel: w390 -> [w407]
                tunnel: [w407] -> w395
                tunnel: [w406] -> w394
                tunnel: [w403] -> w393
                tunnel: [w400] -> w391
                tunnel: w395 -> [w462]
                tunnel: w394 -> [w460]
                tunnel: w393 -> [w459]
                tunnel: [w458] -> w392
                tunnel: w391 -> [w457]
                tunnel: [w534] -> w396
                tunnel: w392 -> [w533]
                frame #0 {
                  n212 = Divide(x=w425, y=i64 1000) -> (x/y=w420:dbl)
                  n213 = local read "BD 1 Frequency 2 (MHz)"() -> (w405:dbl)
                  n214 = Multiply(x="Osc. freq. (Hz)", y=6.283185307179586) -> (x*y=w423:dbl)
                  n215 = Multiply(x=w420, y=w426) -> (x*y=w422:dbl)
                  n216 = Multiply(x=w423, y=w422) -> (x*y=w402:dbl)
                  n217 = local read "BD 1 Frequency 1 (MHz)"() -> (w410:dbl)
                  n218 = local read "BD 2 Frequency 1 (MHz)"() -> (w409:dbl)
                  n219 = case shown="True" w407 {
                    tunnel: w402 -> [w432 w437]
                    tunnel: w410 -> [_ w448]
                    tunnel: w405 -> [_ w449]
                    tunnel: [w429 w443] -> w408
                    tunnel: [FALSE w440] -> w403
                    tunnel: [0.0 w433] -> w400
                    frame False {
                      n220 = Sine(x=w432) -> (sin(x)=w430:dbl)
                      n221 = Multiply(x=w430, y="Osc. amp. (MHz)") -> (x*y=w429:dbl)
                    }
                    frame True {
                      n222 = Cosine(x=w437) -> (cos(x)=w452:dbl)
                      n223 = Subtract(x=w449, y=w448) -> (x-y=w447:dbl)
                      n224 = Decrement(x=w452) -> (x-1=w451:dbl)
                      n225 = Subtract(x=w447, y="Closest Delta (MHz)") -> (x-y=w444:dbl)
                      n226 = Divide(x=w451, y=-2.0) -> (x/y=w445:dbl)
                      n227 = Multiply(x=w445, y=w444) -> (x*y=w443:dbl)
                      n228 = local read "Vec Mean of T1 T2"() -> (w439:dbl[])
                      n229 = Greater?(x=w439, y="Stop F (pN)") -> (0:w441:bool[])
                      n230 = Or Array Elements(Boolean array=w441) -> (logical OR=w440:bool)
                      n231 = Divide(x=w437, y=6.283185307179586) -> (x/y=w436:dbl)
                      n232 = Round Toward +Infinity(x=w436) -> (ceil(x): smallest int >= x=w433:dbl)
                      "Attempts" <- w433
                      n233 = Greater?(x=w433, y="Attempt Limit") -> (0:w435:bool)
                      n234 = case shown="True" w435 {
                        frame False {
                        }
                        frame True {
                          n235 = local write "Fish for Tether"(FALSE ("Fish for Tether")) -> ()
                          n236 = call <vilib>:"Beep.vi"() -> ()  [unwired: 3 in, 9 out]
                          n237 = local read "Messages"() -> (w454:string)
                          n238 = call "Update messages.vi"("Message to add"="Tether fishing timeout." ("Messages"), "Old message string"=w454) -> ("New message string"=→"Messages":string)
                        }
                      }
                    }
                  }
                  n239 = Select(t=w410, s="Scan axis 2", f=w409) -> (s? t:f=w413:dbl)
                  n240 = Add(x=w408, y=w413) -> (x+y=w406:dbl)
                  n241 = Select(t=w406, s="Scan axis 2", f=w410) -> (s? t:f=w416:dbl)
                  n242 = Select(t=w409, s="Scan axis 2", f=w406) -> (s? t:f=w415:dbl)
                  n243 = local read "Y RF Frequency Limits (MHz)"() -> (w411:T16)
                  n244 = local read "X RF Frequency Limits (MHz)"() -> (w412:T16)
                  n245 = local read "BD 1 Frequency 3 (MHz)"() -> (w419:dbl)
                  n246 = local read "BD 2 Frequency 2 (MHz)"() -> (w418:dbl)
                  n247 = local read "BD 2 Frequency 3 (MHz)"() -> (w417:dbl)
                  n248 = call "set RF board frequency - interlace.vi"("Board 2 Frequency Limits"=w411, "Board 1 Frequency Limits"=w412, "FPGA VI Reference In"=w404, "Board 2 Frequency 3 (MHz)"=w417, "Board 1 Frequency 3 (MHz)"=w419, "Board 2 Frequency 2 (MHz)"=w418, "Board 2 Frequency 1 (MHz)"=w415, "Board 1 Frequency 2 (MHz)"=w405, "Board 1 Frequency 1  (MHz)"=w416) -> ()  [unwired: 1 in, 2 out]
                }
                frame #1 {
